vi "Make Protection Signal.vi"(11 "Node Ptr":T1=18446744073709551615 format="%.0x") -> ()   [LabVIEW 2019, in "Protection and Counter Addon System Explorer.lvlib"]
uses:
  Protection and Counter Addon System Explorer.lvlib
  <vilib>/NI VeriStand/Custom Device API/Custom Device Item Ref.ctl
  Addon Shared/SubVIs/GUID Lookup.vi
  Addon Shared/Protection and Counter Addon Shared.lvlib
  SubModules/Frame-Protection-Support/Source/System Explorer/Protection and Counter Support System Explorer.lvlib
  <vilib>/NI VeriStand/Custom Device API/Custom Device API.lvlib
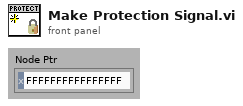
[diagram p1: front panel]
types:
  T1 = typedef "Custom Device API.lvlib/Custom Device Item Ref.ctl" = u64
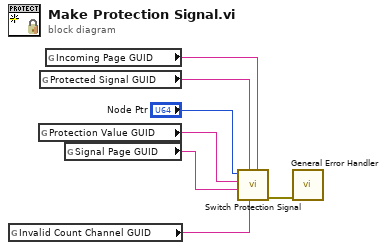
[diagram p0: block diagram]
diagram:
  n1 = global read "GUID Lookup.vi" "Invalid Count Channel GUID"() -> (w2:string)
  n2 = global read "GUID Lookup.vi" "Protection Value GUID"() -> (w5:string)
  n3 = global read "GUID Lookup.vi" "Protected Signal GUID"() -> (w3:string)
  n4 = global read "GUID Lookup.vi" "Incoming Page GUID"() -> (w1:string)
  n5 = global read "GUID Lookup.vi" "Signal Page GUID"() -> (w4:string)
  n6 = call "Switch Protection Signal.vi"("Incoming Page GUID"=w1, "Invalid Count Channel GUID"=w2, "Protected Signal GUID"=w3, "Signal Page GUID"=w4, "Protection Value GUID"=w5, "Node Ptr"="Node Ptr") -> ("error out"=w7:errorcluster)  [unwired: 5 in]
  n7 = call <vilib>:"General Error Handler.vi"("error in (no error)"=w7) -> ()  [unwired: 10 in, 5 out]
